vi "黑白权值.vi"(0 "输入棋盘状态":i32[][](array[numeric]), 2 "初始棋盘权值":sgl[][](array[numeric])) -> (14 "输出棋盘状态":i32[][](array[numeric]), 17 "白子棋盘总权值":sgl[][](array[numeric]), 18 "黑子棋盘总权值":sgl[][](array[numeric]))   [LabVIEW 2018]
panel:
  out "黑棋棋盘权值":sgl[][](array[numeric])
  out "白子棋盘权值":sgl[][](array[numeric])
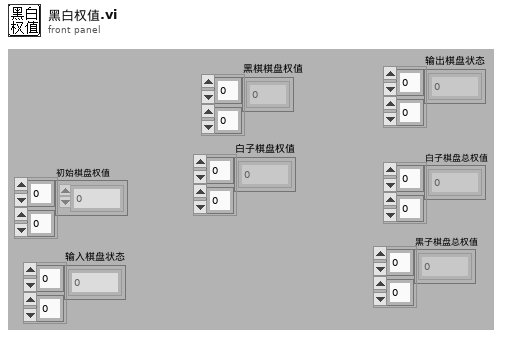
[diagram p1: front panel]
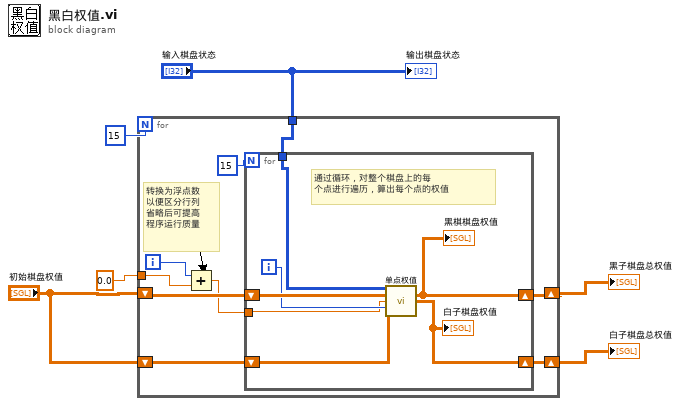
[diagram p0: block diagram]
diagram:
  n1 = for {
    N: 15 -> [_]
    tunnel: "输入棋盘状态" -> [w14]
    shift-right: [w12] -> w3
    shift-left: "初始棋盘权值" -> [w13]
    shift-right: [w11] -> w2
    shift-left: "初始棋盘权值" -> [w10]
    tunnel: sgl 0.0 ("y") -> [w9]
    i -> [w8]
    # "转换为浮点数\n以便区分行列\n省略后可提高\n程序运行质量"
    n2 = Add(x=w8, y=w9) -> (x+y=w7:sgl)
    n3 = for {
      N: 15 -> [_]
      tunnel: w14 -> [w20]
      shift-right: [w21] -> w12
      shift-left: w13 -> [w22]
      shift-right: [w19] -> w11
      shift-left: w10 -> [w18]
      tunnel: w7 -> [w16]
      i -> [w17]
      # "通过循环，对整个棋盘上的每\n个点进行遍历，算出每个点的权值"
      n4 = call "单点权值.vi"("当前棋盘状态"=w20, "黑棋棋盘权值初始"=w22, "行"=w16, "列"=w17, "白棋棋盘权值初始"=w18) -> ("黑子棋盘权值"=w21:sgl[][], "白子棋盘权值"=w19:sgl[][])  [unwired: 8 in, 1 out]
      "黑棋棋盘权值" <- w21
      "白子棋盘权值" <- w19
    }
  }
  "黑子棋盘总权值" <- w3
  "白子棋盘总权值" <- w2
  "输出棋盘状态" <- "输入棋盘状态"
